vi "XML writer.vi"() -> (0 "error out":errorcluster)   [LabVIEW 2014]
uses:
  <vilib>/Utility/sysdir.llb/System Directory Type.ctl
  <vilib>/xml/Load XML File.vi
  <vilib>/xml/Close Reference(Node).vi
  <vilib>/xml/NI_XML.lvlib
  <resource>/objmgr/DOMUserDefRef.rc
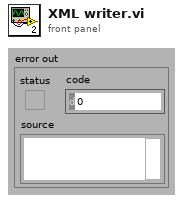
[diagram p1: front panel]
types:
  T1 = typedef "System Directory Type.ctl" = i32
  T2 = enum32{"invalid app kind", "Development System", "Run Time System", "Student Edition", "Embedded LabVIEW", "Evaluation", "Custom"}
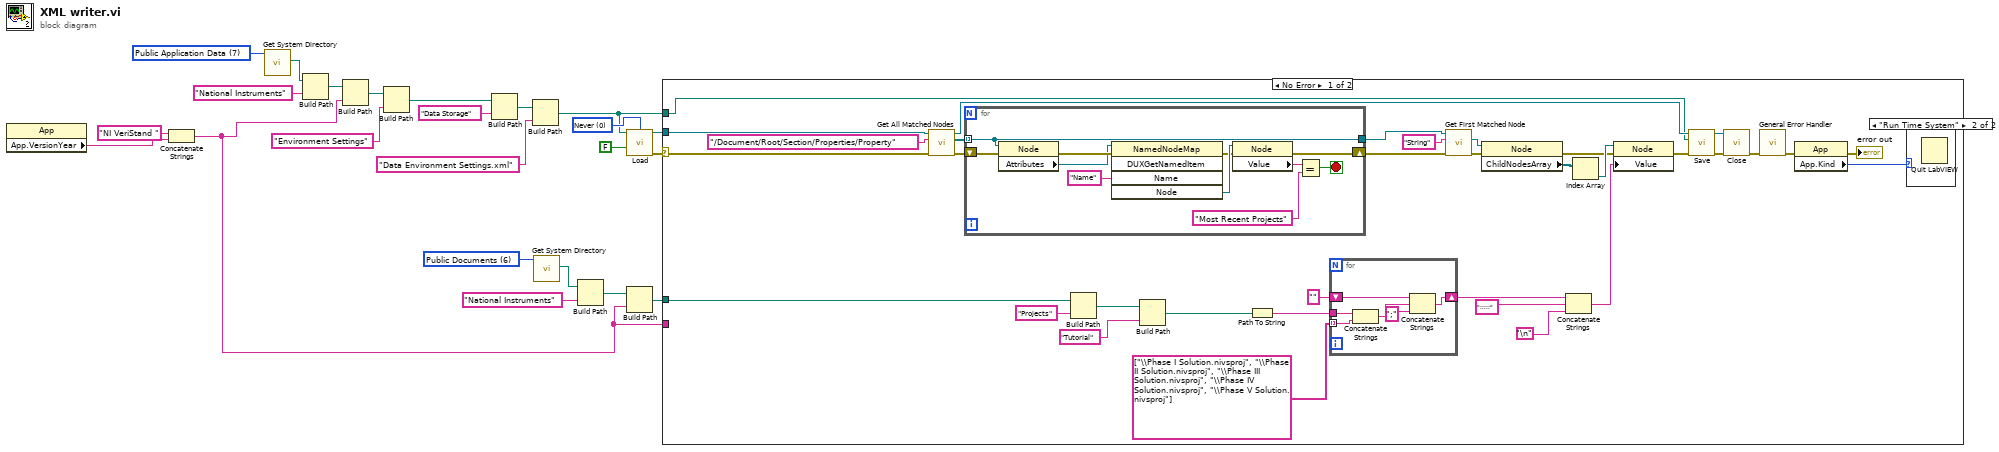
[diagram p0: block diagram]
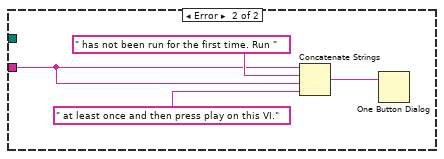
[diagram p3: hidden frame]
diagram:
  w8 = T1 6 items=["User Home", "User Desktop", "User Documents", "User Application Data", "User Preferences", "User Temporary", "Public Documents", "Public Application Data", "Public Preferences", "System Core Libraries", "System Installed Libraries", "Application Files", "Boot Volume Root"] ("system directory type")
  w13 = 0 items=["Never", "Always", "Auto"] ("validate on load (Auto)")
  w20 = T1 7 items=["User Home", "User Desktop", "User Documents", "User Application Data", "User Preferences", "User Temporary", "Public Documents", "Public Application Data", "Public Preferences", "System Core Libraries", "System Installed Libraries", "Application Files", "Boot Volume Root"] ("system directory type")
  n1 = property class="App"() -> ("App.VersionYear"=w2:string)  [unwired: 2 in, 2 out]
  n2 = Concatenate Strings("NI VeriStand " ("string"), w2) -> (w1:string)
  n3 = call <vilib>:"Get System Directory.vi"("system directory type"=w20) -> ("system directory"=w21:path)  [unwired: 10 in]
  n4 = Build Path(base path=w21, name or relative path="National Instruments") -> (appended path=w23:path)
  n5 = Build Path(base path=w23, name or relative path=w1) -> (appended path=w9:path)
  n6 = Build Path(base path=w9, name or relative path="Environment Settings") -> (appended path=w17:path)
  n7 = Build Path(base path=w17, name or relative path="Data Storage") -> (appended path=w15:path)
  n8 = Build Path(base path=w15, name or relative path="Data Environment Settings.xml") -> (appended path=w11:path)
  n9 = call <vilib>:"Get System Directory.vi"("system directory type"=w8) -> ("system directory"=w5:path)  [unwired: 10 in]
  n10 = Build Path(base path=w5, name or relative path="National Instruments") -> (appended path=w6:path)
  n11 = call-poly <vilib>:"Load.vi"("path to XML document"=w11, "validate on load (Auto)"=w13, "load external DTD (True)"=FALSE) -> ("DOM document out"=w12:refnum<k20>, "error out"=w10:errorcluster)  [unwired: 10 in, 1 out]
  n12 = Build Path(base path=w6, name or relative path=w1) -> (appended path=w4:path)
  n13 = case shown="No Error" w10 {
    selector: w10 -> [w28 _]
    tunnel: w12 -> [w46 _]
    tunnel: w11 -> [w29 _]
    tunnel: w4 -> [w27 _]
    tunnel: w1 -> [_ w77]
    frame No Error {
      n14 = call <vilib>:"Get All Matched Nodes.vi"("error in (no error)"=w28, "XPath expression"="/Document/Root/Section/Properties/Property", "node in"=w46) -> ("error out"=w44:errorcluster, "node result array"=w43:refnum<k20>[], "node out"=w31:refnum<k20>)  [unwired: 6 in]
      n15 = for {
        shift-right: [w64] -> w40
        shift-left: w44 -> [w61]
        tunnel: w43 -> [w58] mode=indexing
        tunnel: [w58] -> w42
        stop <- w67 stop-if-true
        n16 = property class="Node"(reference=w58, error in=w61) -> (error out=w62:errorcluster, "Attributes"=w59:refnum<k20>)  [unwired: 1 out]
        n17 = invoke class="NamedNodeMap" method="DUXGetNamedItem"(reference=w59, error in=w62, "Name"="Name") -> (error out=w63:errorcluster, "Node"=w65:refnum<k20>)  [unwired: 2 in, 3 out]
        n18 = property class="Node"(reference=w65, error in=w63) -> (error out=w64:errorcluster, "Value"=w60:string)  [unwired: 1 out]
        n19 = Equal?(x=w60, y="Most Recent Projects") -> (x = y?=w67:bool)
      }
      n20 = Build Path(base path=w27, name or relative path="Projects") -> (appended path=w25:path)
      n21 = Build Path(base path=w25, name or relative path="Tutorial") -> (appended path=w49:path)
      n22 = Path To String(path=w49) -> (string=w48:string)
      n23 = for {
        tunnel: string[] ["\\Phase I Solution.nivsproj", "\\Phase II Solution.nivsproj", "\\Phase III Solution.nivsproj", "\\Phase IV Solution.nivsproj", "\\Phase V Solution.nivsproj"] -> [w73] mode=indexing
        tunnel: w48 -> [w74]
        shift-right: [w69] -> w54
        shift-left: "" -> [w72]
        n24 = Concatenate Strings(w74, w73) -> (w71:string)
        n25 = Concatenate Strings(w72, w71, ";" ("string")) -> (w69:string)
      }
      n26 = call <vilib>:"Get First Matched Node.vi"("error in (no error)"=w40, "XPath expression"="String", "node in"=w42) -> ("error out"=w34:errorcluster, "node result"=w39:refnum<k20>)  [unwired: 6 in, 1 out]
      n27 = property class="Node"(reference=w39, error in=w34) -> (error out=w35:errorcluster, "ChildNodesArray"=w38:refnum<k20>[])  [unwired: 1 out]
      n28 = Concatenate Strings(w54, ";;;;;" ("string"), "\n") -> (w36:string)
      n29 = Index Array(array=w38) -> (element=w37:refnum<k20>)  [unwired: 1 in]
      n30 = property class="Node"(reference=w37, error in=w35, "Value"=w36) -> (error out=w33:errorcluster)  [unwired: 1 out]
      n31 = call <vilib>:"Save.vi"("error in (no error)"=w33, "XML file path"=w29, "DOM document in"=w31) -> ("error out"=w32:errorcluster, "DOM document out"=w30:refnum<k20>)  [unwired: 6 in, 1 out]
      n32 = call-poly <vilib>:"Close.vi"("error in (no error)"=w32, "node"=w30) -> ("error out"=w47:errorcluster)  [unwired: 7 in]
      n33 = call <vilib>:"General Error Handler.vi"("error in (no error)"=w47) -> ("error out"=w51:errorcluster)  [unwired: 10 in, 4 out]
      n34 = property class="App"(error in=w51) -> (error out=→"error out":errorcluster, "App.Kind"=w52:T2)  [unwired: 1 in, 1 out]
      n35 = case shown="\"Run Time System\"" w52 {
        frame "invalid app kind", Default {
        }
        frame "Run Time System" {
          n36 = Quit LabVIEW() -> ()  [unwired: 1 in]
        }
      }
    }
    frame Error {
      n37 = Concatenate Strings(w77, " has not been run for the first time. Run " ("string"), w77, " at least once and then press play on this VI." ("string")) -> (w75:string)
      n38 = One Button Dialog(message=w75) -> ()  [unwired: 1 in, 1 out]
    }
  }
